vi "RSZVB Set Internal Signal Source AUX.vi"(8 "error in (no error)":errorcluster {"code" format="%.0x"}, 9 "Internal Signal Source (0)":i32, 10 "Channel (1)":i32=1, 11 "VISA session":refnum<visa-resource-name>) -> (0 "error out":errorcluster {"code" format="%.0x"}, 3 "dup VISA session":refnum<visa-resource-name>)   [LabVIEW 2011]
doc: "Selects an analyzer port as a signal source for the Aux LO signal in a vector mixer measurement (option R&S ZVA-K5). The Aux LO signal is fed to the MEAS and REF mixers.\n\nRemote-control command(s):\n[SENSe<Ch>:]FREQuency:CONVersion:MIXer:AINTernal NONE | <port_number>"
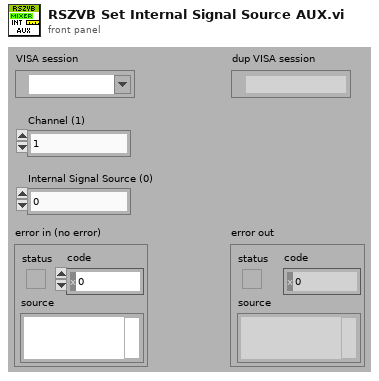
[diagram p1: front panel]
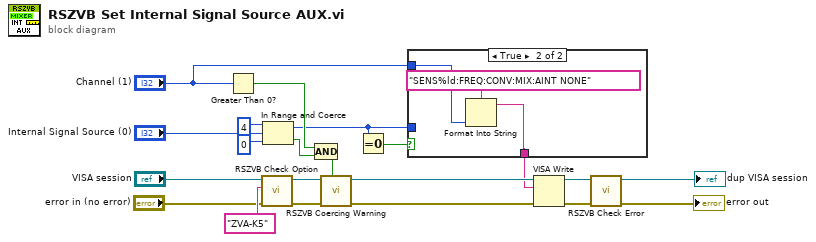
[diagram p0: block diagram]
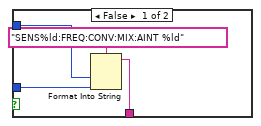
[diagram p2: hidden frame]
diagram:
  n1 = Greater Than 0?(x="Channel (1)") -> (x > 0?=w14:bool)
  n2 = call "RSZVB Check Option.vi"("error in (no error)"="error in (no error)", "Options"="ZVA-K5", "VISA session"="VISA session") -> ("error out"=w1:errorcluster, "dup VISA session"=w2:refnum<visa-resource-name>)  [unwired: 7 in]
  n3 = In Range and Coerce(upper limit=4, x="Internal Signal Source (0)", lower limit=0) -> (coerced(x)=w11:i32, In Range?=w15:bool)
  n4 = Compound Arithmetic op=AND(w14, w15) -> (w13:bool)
  n5 = call "RSZVB Coercing Warning.vi"("In Range?"=w13, "error in (no error)"=w1, "VISA session"=w2) -> ("error out"=w18:errorcluster, "dup VISA session"=w19:refnum<visa-resource-name>)  [unwired: 7 in]
  n6 = Equal To 0?(x=w11) -> (x = 0?=w10:bool)
  n7 = case shown="True" w10 {
    tunnel: [w24 w27] -> w12
    tunnel: w11 -> [w23 _]
    tunnel: "Channel (1)" -> [w22 w26]
    frame False {
      n8 = Format Into String(format string="SENS%ld:FREQ:CONV:MIX:AINT %ld", w22, w23) -> (resulting string=w24:string)  [unwired: 2 in, 1 out]
    }
    frame True {
      n9 = Format Into String(format string="SENS%ld:FREQ:CONV:MIX:AINT NONE", w26) -> (resulting string=w27:string)  [unwired: 2 in, 1 out]
    }
  }
  n10 = VISA Write(VISA resource name=w19, write buffer=w12, error in (no error)=w18) -> (VISA resource name out=w16:refnum<visa-resource-name>, error out=w17:errorcluster)  [unwired: 1 out]
  n11 = call "RSZVB Check Error.vi"("error in (no error)"=w17, "VISA session"=w16) -> ("error out"=→"error out":errorcluster, "dup VISA session"=→"dup VISA session":refnum<visa-resource-name>)  [unwired: 8 in]
